vi "Replace Message Specifier.vi"(11 "format string":string) -> (3 "resulting string":string)   [LabVIEW 2018, in "GLog.lvlib" / "Format String.lvclass"]
uses:
  Format String.lvclass
  <vilib>/regexp/Match Regular Expression.xnode
panel:
  # "Connector Pane"
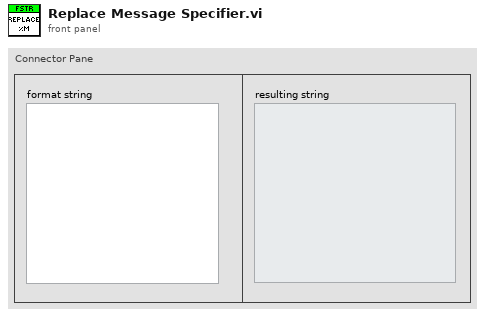
[diagram p1: front panel]
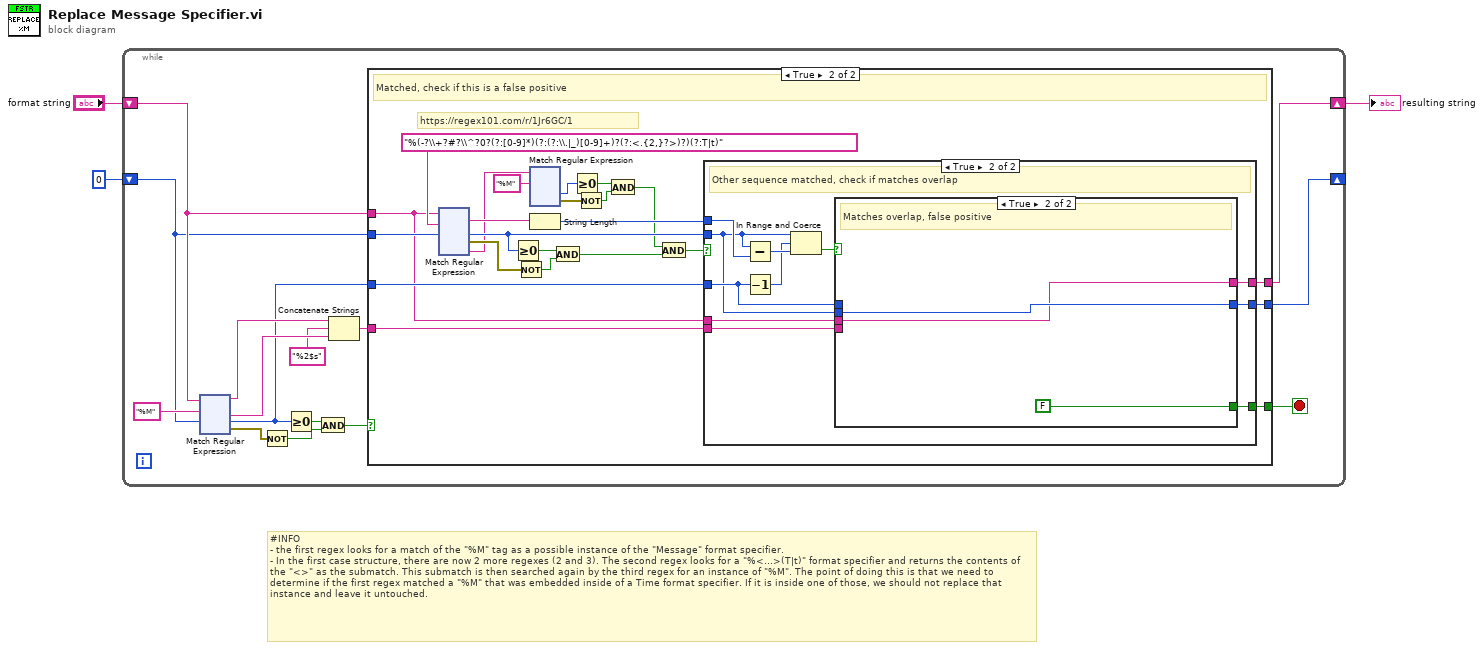
[diagram p0: block diagram]
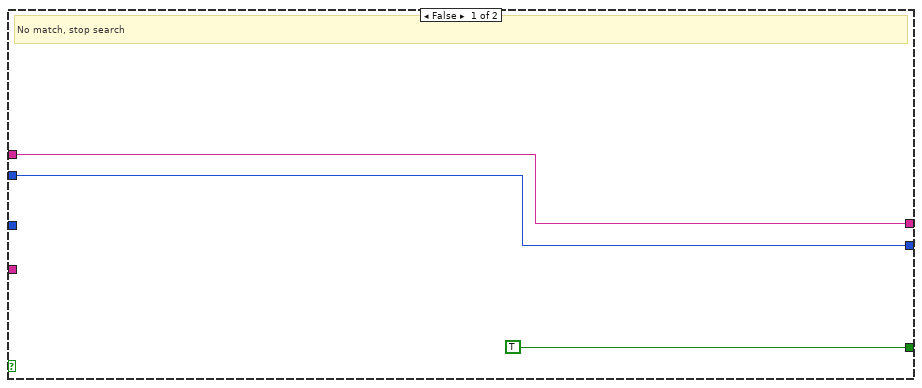
[diagram p2: hidden frame]
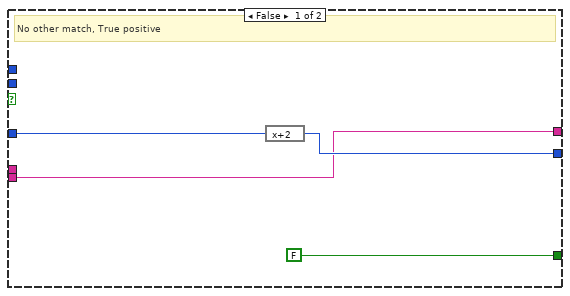
[diagram p3: hidden frame]
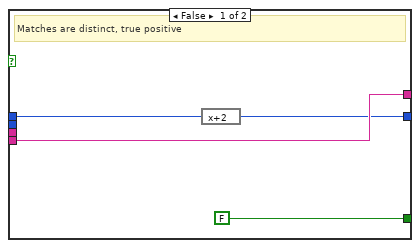
[diagram p4: hidden frame]
diagram:
  # "#INFO\n- the first regex looks for a match of the \"%M\" tag as a possible instance of the \"Message\" format specifier. \n- In the first case structure, there are now 2 more regexes (2 and 3). The second regex looks for a \"%<...>(T|t)\" format specifier and returns the contents of the \"<>\" as the submatch. This submatch is then searched again by the third regex for an instance of \"%M\". The point of doing this is that we need to determine if the first regex matched a \"%M\" that was embedded inside of a Time format specifier. If it is inside one of those, we should not replace that instance and leave it untouched."
  n1 = while {
    shift-right: [w6] -> w2
    shift-left: "format string" -> [w12]
    shift-right: [w5] -> _
    shift-left: 0 ("offset (0)") -> [w11]
    stop <- w7 stop-if-true
    n2 = xnode "Match Regular Expression"("input string"=w12, "regular expression"="%M", "offset (0)"=w11) -> ("before match"=w14:string, "after match"=w13:string, "offset past match"=w8:i32, "error out"=w16:errorcluster)  [unwired: 3 in, 1 out]
    n3 = Not(x=w16) -> (.not. x?=w15:bool)
    n4 = Greater Or Equal To 0?(x=w8) -> (x >= 0?=w17:bool)
    n5 = And(x=w17, y=w15) -> (x .and. y?=w9:bool)
    n6 = Concatenate Strings(w14, "%2$s" ("string"), w13) -> (w4:string)
    n7 = case shown="True" w9 {
      tunnel: w12 -> [w20 w33]
      tunnel: w11 -> [w19 w44]
      tunnel: w8 -> [_ w37]
      tunnel: [TRUE w32] -> w7
      tunnel: [w20 w34] -> w6
      tunnel: [w19 w36] -> w5
      tunnel: w4 -> [_ w35]
      frame False {
        # "No match, stop search"
      }
      frame True {
        # "https://regex101.com/r/1Jr6GC/1"
        # "Matched, check if this is a false positive"
        n8 = xnode "Match Regular Expression"("input string"=w33, "regular expression"="%(-?\\+?#?\\^?0?(?:[0-9]*)(?:(?:\\.|_)[0-9]+)?(?:<.{2,}?>)?)(?:T|t)", "offset (0)"=w44) -> ("whole match"=w31:string, "offset past match"=w39:i32, "error out"=w40:errorcluster, "submatch 1"=w22:string)  [unwired: 3 in, 2 out]
        n9 = Greater Or Equal To 0?(x=w39) -> (x >= 0?=w41:bool)
        n10 = Not(x=w40) -> (.not. x?=w42:bool)
        n11 = xnode "Match Regular Expression"("input string"=w22, "regular expression"="%M") -> ("offset past match"=w27:i32, "error out"=w26:errorcluster)  [unwired: 4 in, 3 out]
        n12 = String Length(string=w31) -> (length=w38:i32)
        n13 = And(x=w41, y=w42) -> (x .and. y?=w24:bool)
        n14 = Greater Or Equal To 0?(x=w27) -> (x >= 0?=w29:bool)
        n15 = Not(x=w26) -> (.not. x?=w28:bool)
        n16 = And(x=w29, y=w28) -> (x .and. y?=w23:bool)
        n17 = And(x=w23, y=w24) -> (x .and. y?=w25:bool)
        n18 = case shown="True" w25 {
          tunnel: w39 -> [_ w287]
          tunnel: w38 -> [_ w295]
          tunnel: w37 -> [w283 w290]
          tunnel: [w284 w291] -> w36
          tunnel: w35 -> [w282 w288]
          tunnel: [w282 w289] -> w34
          tunnel: w33 -> [_ w286]
          tunnel: [FALSE w285] -> w32
          frame False {
            # "No other match, True positive"
            n19 = expression code="x+2"(w283) -> (w284:i32)
          }
          frame True {
            # "Other sequence matched, check if matches overlap"
            n20 = Subtract(x=w287, y=w295) -> (x-y=w294:i32)
            n21 = Decrement(x=w290) -> (x-1=w293:i32)
            n22 = In Range and Coerce(upper limit=w287, x=w293, lower limit=w294) -> (In Range?=w292:bool)  [unwired: 1 out]
            n23 = case shown="True" w292 {
              tunnel: [w297 w302] -> w291
              tunnel: w290 -> [w299 _]
              tunnel: [w298 w301] -> w289
              tunnel: w288 -> [w298 _]
              tunnel: w287 -> [_ w302]
              tunnel: w286 -> [_ w301]
              tunnel: [FALSE FALSE] -> w285
              frame False {
                # "Matches are distinct, true positive"
                n24 = expression code="x+2"(w299) -> (w297:i32)
              }
              frame True {
                # "Matches overlap, false positive"
              }
            }
          }
        }
      }
    }
  }
  "resulting string" <- w2
